vi "write parameters in a cluster to configuration file.vi"(6 "error in (no error)":errorcluster, 7 "Control in":refnum<vi>, 8 "section":string, 9 "refnum":T1) -> (0 "error out":errorcluster, 3 "refnum out":T1)   [LabVIEW 2015]
uses:
  <vilib>/Utility/config.llb/Config Data RefNum.ctl
  <vilib>/Utility/config.llb/Write Key (Double).vi
  <vilib>/Utility/config.llb/Write Key (String).vi
  <vilib>/Utility/config.llb/Write Key (Boolean).vi
  <vilib>/Utility/config.llb/NI_LVConfig.lvlib
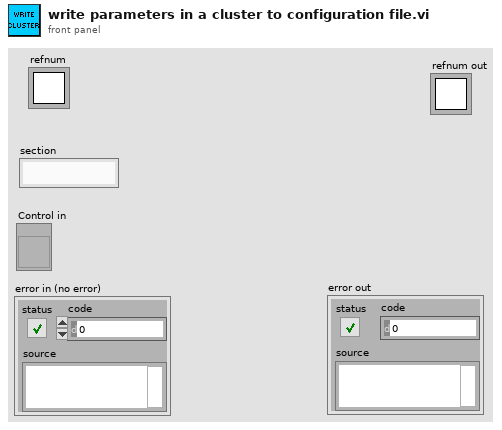
[diagram p1: front panel]
types:
  T1 = typedef "NI_LVConfig.lvlib/Config Data RefNum.ctl" = refnum<k1>
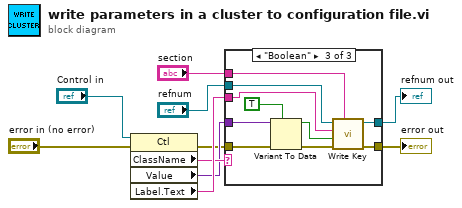
[diagram p0: block diagram]
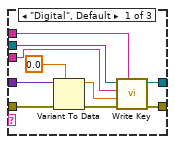
[diagram p2: hidden frame]
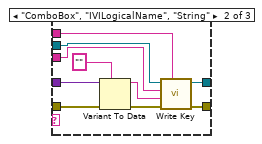
[diagram p3: hidden frame]
diagram:
  n1 = property class="Ctl"(reference="Control in", error in="error in (no error)") -> (error out=w3:errorcluster, "ClassName"=w7:string, "Value"=w6:variant, "Label.Text"=w8:string)  [unwired: 1 out]
  n2 = case shown="\"Boolean\"" w7 {
    tunnel: w6 -> [w20 w30 w40]
    tunnel: w8 -> [w17 w28 w37]
    tunnel: "refnum" -> [w16 w27 w36]
    tunnel: "section" -> [w15 w26 w35]
    tunnel: [w14 w25 w31] -> w1
    tunnel: [w13 w24 w34] -> w4
    tunnel: w3 -> [w12 w23 w32]
    frame "Digital", Default {
      n3 = Variant To Data(error in=w12, type=0.0, Variant=w20) -> (data=w18:dbl, error out=w11:errorcluster)
      n4 = call-poly <vilib>:"Write Key.vi"("section"=w15, "error in (no error)"=w11, "value"=w18, "key"=w17, "refnum"=w16) -> ("error out"=w13:errorcluster, "refnum out"=w14:T1)  [unwired: 4 in, 1 out]
    }
    frame "ComboBox", "IVILogicalName", "String" {
      n5 = Variant To Data(error in=w23, type="", Variant=w30) -> (data=w29:string, error out=w22:errorcluster)
      n6 = call-poly <vilib>:"Write Key.vi"("section"=w26, "error in (no error)"=w22, "value"=w29, "key"=w28, "refnum"=w27) -> ("error out"=w24:errorcluster, "refnum out"=w25:T1)  [unwired: 4 in, 1 out]
    }
    frame "Boolean" {
      n7 = Variant To Data(error in=w32, type=TRUE, Variant=w40) -> (data=w38:bool, error out=w33:errorcluster)
      n8 = call-poly <vilib>:"Write Key.vi"("section"=w35, "error in (no error)"=w33, "value"=w38, "key"=w37, "refnum"=w36) -> ("error out"=w34:errorcluster, "refnum out"=w31:T1)  [unwired: 4 in, 1 out]
    }
  }
  "error out" <- w4
  "refnum out" <- w1
